vi "Initialize Thread.vi"(7 "component name":string, 8 "error in (no error)":errorcluster, 10 "Thread Configuration":refnum<class "Thread Configuration.lvclass">, 11 "UDP Transceiver in":refnum<class "UDP Transceiver.lvclass">) -> (0 "error out":errorcluster, 3 "UDP Transceiver out":refnum<class "UDP Transceiver.lvclass">)   [LabVIEW 2023, in "UDP.lvlib" / "UDP Transceiver.lvclass"]
uses:
  UDP Transceiver.lvclass
  Users/Public/Documents/National Instruments/NI VeriStand 2023/Custom Devices/Data Sharing Framework/Linux_x64/DSF Core.lvlibp/Classes/Configuration/Core/Thread/Thread Configuration.lvclass
  C:/Users/Public/Documents/National Instruments/NI VeriStand 2023/Custom Devices/Data Sharing Framework/Linux_x64/DSF Core.lvlibp/Classes/Configuration/Core/Core Configuration.lvclass
  Configuration/Thread/UDP Thread Configuration.lvclass
  UDP Transceiver.lvclass/UDP Transceiver.ctl
  Users/Public/Documents/National Instruments/NI VeriStand 2023/Custom Devices/Data Sharing Framework/Linux_x64/DSF Core.lvlibp/Classes/Configuration/Core/Core Configuration.lvclass
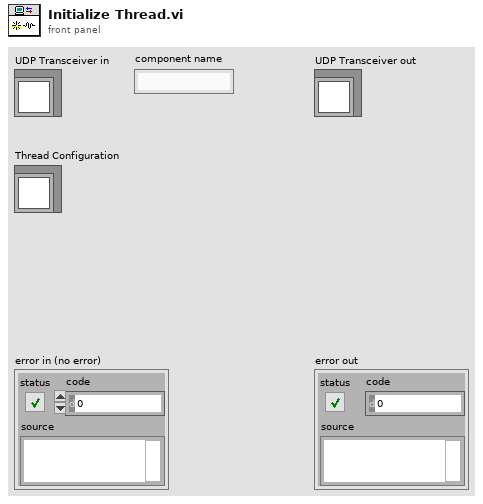
[diagram p1: front panel]
types:
  T1 = typedef "DSF Core.lvlibp/DSF Settings Info.ctl" = cluster{"component":string, "values":cluster{"key":string, "value":string}[]}
  T2 = typedef "UDP.lvlib/UDP Thread Configuration.lvclass/Thread Settings.ctl" = cluster{"local port":u16, "local address":u32}
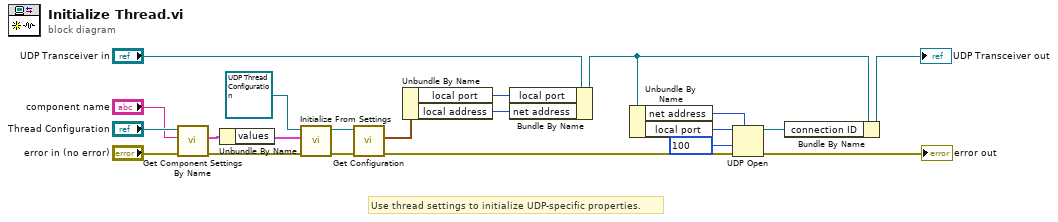
[diagram p0: block diagram]
diagram:
  # "Use thread settings to initialize UDP-specific properties."
  n1 = call "Get Component Settings By Name.vi"("error in (no error)"="error in (no error)", "component name"="component name", "Runtime Configuration in"="Thread Configuration") -> ("error out"=w9:errorcluster, "component settings"=w15:T1)  [unwired: 6 in, 1 out]
  n2 = Unbundle By Name(w15) -> ("values"=w14:cluster{"key":string, "value":string}[])
  n3 = call-dynamic "Initialize From Settings.vi"("error in (no error)"=w9, "settings"=w14, "UDP Thread Configuration in"=refnum<class "UDP Thread Configuration.lvclass"> refnum) -> ("error out"=w7:errorcluster, "UDP Thread Configuration out"=w8:refnum<class "UDP Thread Configuration.lvclass">)  [unwired: 7 in]
  n4 = call "Get Configuration.vi"("error in (no error)"=w7, "DSF UDP Thread Configuration in"=w8) -> ("error out"=w1:errorcluster, "thread settings"=w6:T2)  [unwired: 7 in, 1 out]
  n5 = Unbundle By Name(w6) -> ("local port"=w2:u16, "local address"=w3:u32)
  n6 = Bundle By Name(cluster="UDP Transceiver in", "local port"=w2, "net address"=w3) -> (w4:refnum<class "UDP Transceiver.lvclass">)
  n7 = Unbundle By Name(w4) -> ("net address"=w18:u32, "local port"=w21:u16)
  n8 = UDP Open(7:w18, 8:w1, 9:100 ("timeout ms (25000)"), 11:w21) -> (port=w19:refnum<k16>, 0:→"error out":errorcluster)  [unwired: 1 in, 1 out]
  n9 = Bundle By Name(cluster=w4, "connection ID"=w19) -> (→"UDP Transceiver out":refnum<class "UDP Transceiver.lvclass">)
